vi "build-base-paths.vi"(6 "parent-subfolder-name":string="parents", 8 "error in":errorcluster, 10 "dest-subfolder":string, 11 "input-file":path) -> (0 "error out":errorcluster, 2 "input-file-name":string, 3 "Destination Path":path)   [LabVIEW 2017]
uses:
  <vilib>/Utility/error.llb/DialogType.ctl
  labview/utils_lib/utils.lvlib
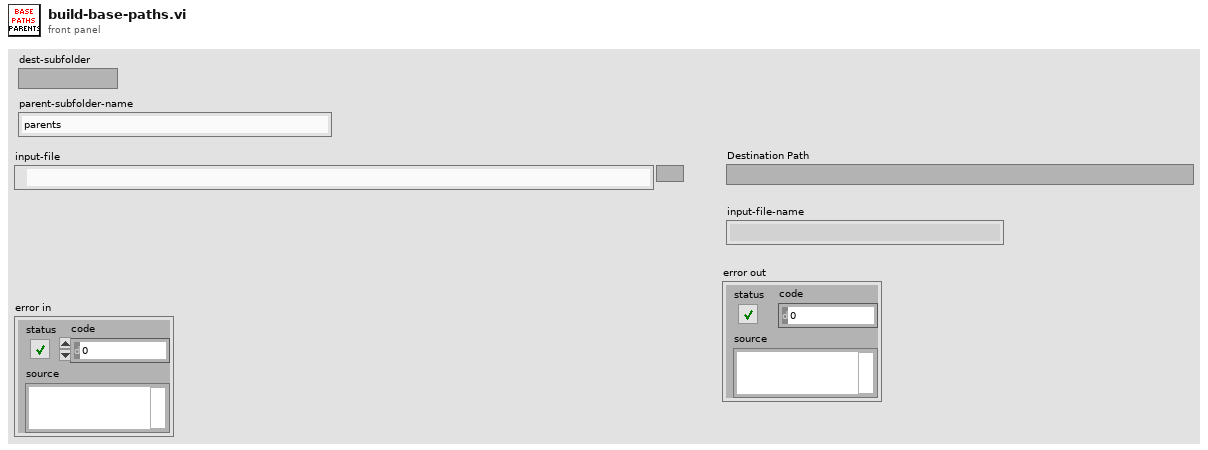
[diagram p1: front panel]
types:
  T1 = typedef "DialogType.ctl" = u16
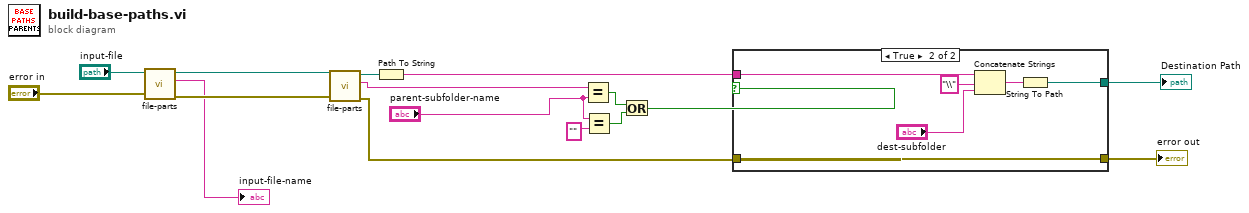
[diagram p0: block diagram]
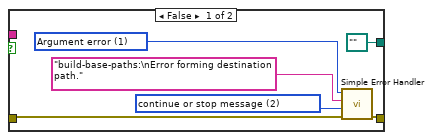
[diagram p2: hidden frame]
diagram:
  n1 = call "file-parts.vi"("error in"="error in", "full-path-file"="input-file") -> ("error out"=w14:errorcluster, "file-name"=→"input-file-name":string, "path-root"=w15:path)  [unwired: 7 in]
  n2 = call "file-parts.vi"("error in"=w14, "full-path-file"=w15) -> ("error out"=w2:errorcluster, "file-name"=w9:string, "path-root"=w11:path)  [unwired: 7 in]
  n3 = Path To String(path=w11) -> (string=w10:string)
  n4 = Equal?(x=w9, y="parent-subfolder-name") -> (x = y?=w6:bool)
  n5 = Equal?(x="parent-subfolder-name", y="") -> (x = y?=w5:bool)
  n6 = Or(x=w6, y=w5) -> (x .or. y?=w4:bool)
  n7 = case shown="True" w4 {
    tunnel: w10 -> [_ w28]
    tunnel: [path "" w25] -> w3
    tunnel: w2 -> [w20 w24]
    tunnel: [w21 w24] -> w1
    frame False {
      w17 = 1 items=["No error", "Argument error", "Memory is full", "Out of zone", "End of file", "File already open", "Generic file I/O error", "File not found", "File permission error", "Disk is full", "Duplicate path", "Too many files open", "System feature not enabled", "Resource file not found", "Cannot add resource", "Resource not found", "Image not found", "Image memory error", "Pen does not exist", "Config type invalid", "Config token not found", "Config parse error", "Config memory error", "Bad external code format", "Bad external code offset", "External code not present", "Null window", "Destroy window error", "Null menu", "Print aborted", "Bad print record", "Print driver error", "Windows error during printing", "Memory error during printing", "Print dialog error", "Generic print error", "Invalid device refnum", "Device not found", "Device parameter error", "Device unit error", "Cannot open device", "Device call aborted", "Generic error", "Cancelled by user", "Object ID too low", "Object ID too high", "Object not in heap", "Unknown heap", "Unknown object (invalid DefProc)", "Unknown object (DefProc not in table)", "Message out of range", "Invalid (null) method", "Unknown message", "Manager call not supported", "Bad address", "Network operation in progress", "Network operation timed out", "Connection is busy", "Network attribute not supported", "Network error", "Address in use", "System out of memory", "Connection aborted", "Connection refused", "Not connected", "Already connected", "Connection closed", "Initialization error (interapplication manager)", "Bad occurrence", "Wait on unbound occurrence handler", "Occurrence queue overflow", "Datalog type conflict", "Unused", "Unrecognized type (interapplication manager)", "Memory corrupt", "Failed to make temporary DLL", "Old CIN version", "Drag socket not found", "Failed to load drop-object", "Failed to register OLE object", "Failed to release OLE object", "Format specifier type mismatch", "Unknown format specifier", "Too few format specifiers", "Too many format specifiers", "Scan failed", "Newer CIN version", "Error converting to variant", "Runtime menu error", "Password tampered", "Variant attribute not found", "Incompatible variant data type", "Event data is not available", "Event Store is not present", "Occurrence is not found", "Event Queue is not created", "Event info is not available", "Refnum passed is NULL", "Error retrieving Class GUID", "Error retrieving CoClass GUID", "Error retrieving TypeLib GUID.", "Bad built application magic bytes.", "Specific driver is different from the specific driver associated with the Logical Name.", "There is no session opened to the class driver.", "Max Error", "MAX - Error with config objects", "MAX - Error loading configuration", "MAX - Group not supported"]
      w19 = T1 2 items=["no dialog", "OK message", "continue or stop message", "OK message + warnings", "continue/stop + warnings"] ("type of dialog (OK msg:1)")
      n8 = call <vilib>:"Simple Error Handler.vi"("error code (no error:0)"=w17, "error source (\" \")"="build-base-paths:\nError forming destination path." ("error source (\" \")"), "type of dialog (OK msg:1)"=w19, "error in (no error)"=w20) -> ("error out"=w21:errorcluster)  [unwired: 1 in, 4 out]
    }
    frame True {
      n9 = Concatenate Strings(w28, "\\", "dest-subfolder") -> (w26:string)
      n10 = String To Path(string=w26) -> (path=w25:path)
    }
  }
  "error out" <- w1
  "Destination Path" <- w3
